vi "Instruments.vi"(0 "task in":refnum<k21>, 1 "Error In":errorcluster, 2 "Spark":bool, 3 "Mix Fan":bool, 4 "Camera":bool) -> (15 "Error Out":errorcluster, 16 "Tube Inlet State":bool caption="Spark State", 17 "Mix Inlet State":bool caption="Mix Fan State", 18 "Mix Outlet State":bool caption="Camera State")   [LabVIEW 2018]
uses:
  <vilib>/DAQmx/write.llb/DAQmx Write (Digital 1D Bool 1Chan 1Samp).vi
  <vilib>/DAQmx/create/channels.llb/DAQmx Create Channel (DO-Digital Output).vi
  <vilib>/DAQmx/miscellaneous.llb/DAQmx Fill In Error Info.vi
panel:
  # "Instruments"
  # "TRUE:    Activated\nFALSE:  Deactivated"
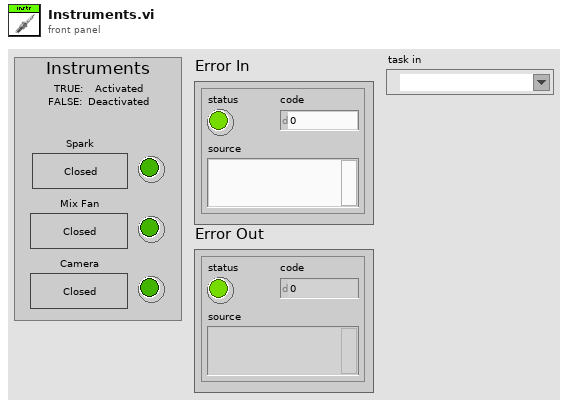
[diagram p1: front panel]
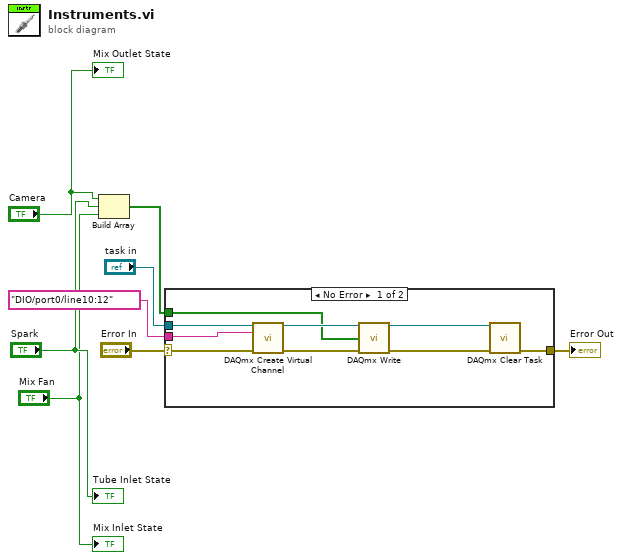
[diagram p0: block diagram]
diagram:
  n1 = Build Array("Camera", "Spark", "Mix Fan") -> (w5:bool[])
  n2 = case shown="No Error" "Error In" {
    selector: "Error In" -> [w13 w18]
    tunnel: [w9 w18] -> w7
    tunnel: tag "DIO/port0/line10:12" ("lines") -> [w17 _]
    tunnel: w5 -> [w14 _]
    tunnel: "task in" -> [w12 _]
    frame No Error {
      n3 = call-poly <vilib>:"DAQmx Create Virtual Channel.vi"("task in"=w12, "lines"=w17, "error in"=w13) -> ("task out"=w16:refnum<k21>, "error out"=w15:errorcluster)  [unwired: 11 in]
      n4 = call-poly <vilib>:"DAQmx Write.vi"("task/channels in"=w16, "data"=w14, "error in"=w15) -> ("task out"=w10:refnum<k21>, "error out"=w11:errorcluster)  [unwired: 10 in, 1 out]
      n5 = call <vilib>:"DAQmx Clear Task.vi"("task in"=w10, "error in"=w11) -> ("error out"=w9:errorcluster)  [unwired: 13 in]
    }
    frame Error {
    }
  }
  "Error Out" <- w7
  "Tube Inlet State" <- "Spark"
  "Mix Inlet State" <- "Mix Fan"
  "Mix Outlet State" <- "Camera"
